vi "actuate_gapFreeExp_v0.04.vi"(0 "Phase Cluster":T3, 1 "valve Time Cluster":T2, 2 "Didn't Lift?":bool, 3 "data in":T4={"daq_ao 1"="Dev1/ao0", "daq_ai 1"="Dev1/ai0", "experiment day folder"=path "D:/DATA/8-27-15 save func testing/test.lvm", "Multiclamp init error"=0, "Multiclamp Handle Out"=0, "sampling rate (Hz)"=10000, "trial name"=""}, 5 "PhaseLetter":string, 7 "controls array in":refnum<vi>[](array[refnum]), 9 "time to wait for solution change (min)":dbl=2.5 min=0.0 step=0.01, 11 "error in":errorcluster, 12 "common cluster":T6, 13 "individual controls in":T5) -> (4 "output cluster":T1, 8 "jumptestMonitor":waveform(dbl)[](graph) caption="protocol response", 10 "control array out":refnum<vi>[](array[refnum]), 14 "experiment VI ref":refnum<vi>, 15 "error out":errorcluster)   [LabVIEW 2019]
uses:
  pipette cleaning/pressure box/cleaning_soft/controls/actuator_type.ctl
  pipette cleaning/pressure box/cleaning_soft/controls/actuator_cluster.ctl
  machine_vision/coordinate model vis/transform_properties_actuators.ctl
  machine_vision/controls/transform_cluster_actuator.ctl
  controls/NH_method.ctl
  pipette cleaning/pressure box/cleaning_soft/controls/pressure_box_type.ctl
  pipette cleaning/pressure box/cleaning_soft/controls/pressure_box_control.ctl
  multipatch/controls/multipatch_common_controls_v4.ctl
  controls/memtest_def.ctl
  multipatch/controls/multipatch_individual_controls_v5.ctl
  Controls/Data.ctl
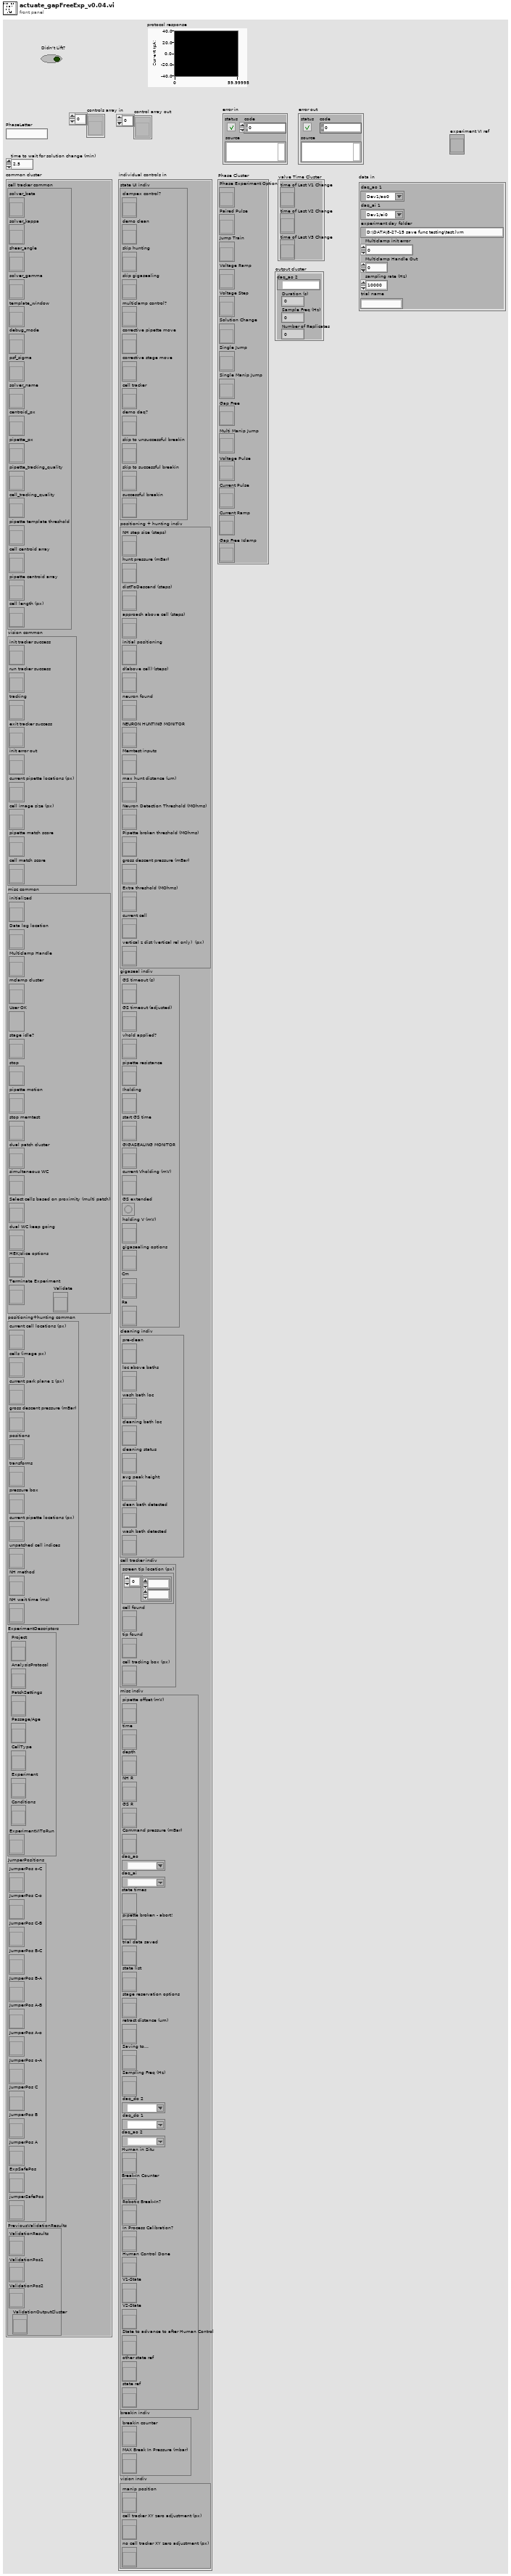
[diagram p1: front panel]
types:
  T1 = cluster{"daq_ao 2":tag, "Duration (s)":dbl, "Sample Freq (Hz)":dbl, "Number of Replicates":i16}
  T2 = cluster{"time of Last V1 Change":refnum<vi>, "time of Last V2 Change":refnum<vi>, "time of Last V3 Change":refnum<vi>}
  T3 = cluster{"Phase Experiment Option":refnum<vi>, "Paired Pulse":refnum<vi>, "Jump Train":refnum<vi>, "Voltage Ramp":refnum<vi>, "Voltage Step":refnum<vi>, "Solution Change":refnum<vi>, "Single Jump":refnum<vi>, "Single Manip Jump":refnum<vi>, "Gap Free":refnum<vi>, "Multi Manip Jump":refnum<vi>, "Voltage Pulse":refnum<vi>, "Current Pulse":refnum<vi>, "Current Ramp":refnum<vi>, "Gap Free Iclamp":refnum<vi>}
  T4 = typedef "Data.ctl" = cluster{"daq_ao 1":tag, "daq_ai 1":tag, "experiment day folder":path, "Multiclamp init error":i32, "Multiclamp Handle Out":u32, "sampling rate (Hz)":i32, "trial name":string}
  T5 = typedef "multipatch_individual_controls_v5.ctl" = cluster{"state UI indiv":cluster{"clampex control?":refnum<vi>, "demo clean":refnum<vi>, "skip hunting":refnum<vi>, "skip gigasealing":refnum<vi>, "multiclamp control?":refnum<vi>, "corrective pipette move":refnum<vi>, "corrective stage move":refnum<vi>, "cell tracker":refnum<vi>, "demo daq?":refnum<vi>, "skip to unsuccessful breakin":refnum<vi>, "skip to successful breakin":refnum<vi>, "successful breakin":refnum<vi>}, "positioning + hunting indiv":cluster{"NH step size (steps)":refnum<vi>, "hunt pressure (mBar)":refnum<vi>, "distToDescend (steps)":refnum<vi>, "approach above cell (steps)":refnum<vi>, "initial positioning":refnum<vi>, "d(above cell) (steps)":refnum<vi>, "neuron found":refnum<vi>, "NEURON HUNTING MONITOR":refnum<vi>, "Memtest inputs":refnum<vi>, "max hunt distance (um)":refnum<vi>, "Neuron Detection Threshold (MOhms)":refnum<vi>, "Pipette broken threshold (MOhms)":refnum<vi>, "gross descent pressure (mBar)":refnum<vi>, "Extra threshold (MOhms)":refnum<vi>, "current cell":refnum<vi>, "vertical z dist (vertical rel only)  (px)":refnum<vi>}, "gigaseal indiv":cluster{"GS timeout (s)":refnum<vi>, "GS timeout (adjusted)":refnum<vi>, "vhold applied?":refnum<vi>, "pipette resistance":refnum<vi>, "Iholding":refnum<vi>, "start GS time":refnum<vi>, "GIGASEALING MONITOR":refnum<vi>, "current Vholding (mV)":refnum<vi>, "GS extended":refnum<vi>, "holding V (mV)":refnum<vi>, "gigasealing options":refnum<vi>, "Cm":refnum<vi>, "Ra ":refnum<vi>}, "cleaning indiv":cluster{"pre-clean":refnum<vi>, "loc above baths":refnum<vi>, "wash bath loc":refnum<vi>, "cleaning bath loc":refnum<vi>, "cleaning status":refnum<vi>, "avg peak height":refnum<vi>, "clean bath detected":refnum<vi>, "wash bath detected":refnum<vi>}, "cell tracker indiv":cluster{"screen tip location (px)":refnum<vi>, "cell found":refnum<vi>, "tip found":refnum<vi>, "cell tracking box (px)":refnum<vi>}, "misc indiv":cluster{"pipette offset (mV)":refnum<vi>, "time":refnum<vi>, "depth":refnum<vi>, "NH R":refnum<vi>, "GS R":refnum<vi>, "Command pressure (mBar)":refnum<vi>, "daq_ao":tag, "daq_ai":tag, "state times":refnum<vi>, "pipette broken - abort!":refnum<vi>, "trial data saved":refnum<vi>, "state list":refnum<vi>, "stage reservation options":refnum<vi>, "retract distance (um)":refnum<vi>, "Saving to...":refnum<vi>, "Sampling Freq (Hz)":refnum<vi>, "daq_do 2":tag, "daq_do 1":tag, "daq_ao 2":tag, "Human in Situ":refnum<vi>, "Break-In Counter":refnum<vi>, "Robotic Break-In?":refnum<vi>, "In Process Calibration?":refnum<vi>, "Human Control Done":refnum<vi>, "V1-State":refnum<vi>, "V2-State":refnum<vi>, "State to advance to after Human Control":refnum<vi>, "other state ref":refnum<vi>, "state ref":refnum<vi>}, "breakin indiv":cluster{"breakin counter":refnum<vi>, "MAX Break In Pressure (mbar)":refnum<vi>}, "vision indiv":cluster{"manip position":refnum<vi>, "cell tracker XY zero adjustment (px)":refnum<vi>, "no cell tracker XY zero adjustment (px)":refnum<vi>}}
  T6 = typedef "multipatch_common_controls_v4.ctl" = cluster{"cell tracker common":cluster{"solver_beta":refnum<vi>, "solver_kappa":refnum<vi>, "shear_angle":refnum<vi>, "solver_gamma":refnum<vi>, "template_window":refnum<vi>, "debug_mode":refnum<vi>, "psf_sigma":refnum<vi>, "solver_name":refnum<vi>, "centroid_px":refnum<vi>, "pipette_px":refnum<vi>, "pipette_tracking_quality":refnum<vi>, "cell_tracking_quality":refnum<vi>, "pipette template threshold":refnum<vi>, "cell centroid array":refnum<vi>, "pipette centroid array":refnum<vi>, "cell length (px)":refnum<vi>}, "vision common":cluster{"init tracker success":refnum<vi>, "run tracker success":refnum<vi>, "tracking":refnum<vi>, "exit tracker success":refnum<vi>, "init error out":refnum<vi>, "current pipette locations (px)":refnum<vi>, "cell image size (px)":refnum<vi>, "pipette match score":refnum<vi>, "cell match score":refnum<vi>}, "misc common":cluster{"initialized":refnum<vi>, "Data log location":refnum<vi>, "Multiclamp Handle":refnum<vi>, "mclamp cluster":refnum<vi>, "User OK":refnum<vi>, "stage idle?":refnum<vi>, "stop":refnum<vi>, "pipette motion":refnum<vi>, "stop memtest":refnum<vi>, "dual patch cluster":refnum<vi>, "simultaneous WC":refnum<vi>, "Select cells based on proximity (multi patch)":refnum<vi>, "dual WC keep going":refnum<vi>, "HEK/slice options":refnum<vi>, "Terminate Experiment":refnum<vi>, "Validate":refnum<vi>}, "positioning+hunting common":cluster{"current cell locations (px)":refnum<vi>, "cells (image px)":refnum<vi>, "current park plane z (px)":refnum<vi>, "gross descent pressure (mBar)":refnum<vi>, "positions":refnum<vi>, "transforms":refnum<vi>, "pressure box":refnum<vi>, "current pipette locations (px)":refnum<vi>, "unpatched cell indices":refnum<vi>, "NH method":refnum<vi>, "NH wait time (ms)":refnum<vi>}, "ExperimentDescriptors":cluster{"Project":refnum<vi>, "AnalysisProtocol":refnum<vi>, "PatchSettings":refnum<vi>, "Passage/Age":refnum<vi>, "CellType":refnum<vi>, "Experiment":refnum<vi>, "Conditions":refnum<vi>, "ExperimentVIToRun":refnum<vi>}, "JumperPositions":cluster{"JumperPos o-C":refnum<vi>, "JumperPos C-o":refnum<vi>, "JumperPos C-B":refnum<vi>, "JumperPos B-C":refnum<vi>, "JumperPos B-A":refnum<vi>, "JumperPos A-B":refnum<vi>, "JumperPos A-o":refnum<vi>, "JumperPos o-A":refnum<vi>, "JumperPos C":refnum<vi>, "JumperPos B":refnum<vi>, "JumperPos A":refnum<vi>, "ExpSafePos":refnum<vi>, "jumperSafePos":refnum<vi>}, "PreviousValidationResults":cluster{"ValidationResults":refnum<vi>, "ValidationPos1":refnum<vi>, "ValidationPos2":refnum<vi>, "ValidationOutputCluster":refnum<vi>}}
  T7 = cluster{"Which Position to use for Experiment":enum16{"Jumper Safe Position", "Experiment Safe Position", "Jumper Position A", "Jumper Position B", "Jumper Position C", "Jumper Position o-A", "Jumper Position A-o", "Jumper Position A-B", "Jumper Position B-A", "Jumper Position B-C", "Jumper Position C-B", "Jumper Position C-o", "Jumper Position o-C", "Don't Move"}, "Duration (s)":dbl, "Valve 1 Position":i16, "Valve 2 Position":i16, "Replicates":dbl, "Vholding (mV)":dbl, "Valve 3 Position":i16, "valve 1 used now?":bool, "valve 2 used now?":bool, "valve 3 used now? ":bool, "Record During Solution Change?":bool}
  T8 = enum16{"Jumper Safe Position", "Experiment Safe Position", "Jumper Position A", "Jumper Position B", "Jumper Position C", "Jumper Position o-A", "Jumper Position A-o", "Jumper Position A-B", "Jumper Position B-A", "Jumper Position B-C", "Jumper Position C-B", "Jumper Position C-o", "Jumper Position o-C", "Don't Move"}
  T9 = enum16{"manipulator 1", "manipulator 2", "manipulator 3", "manipulator 4"}
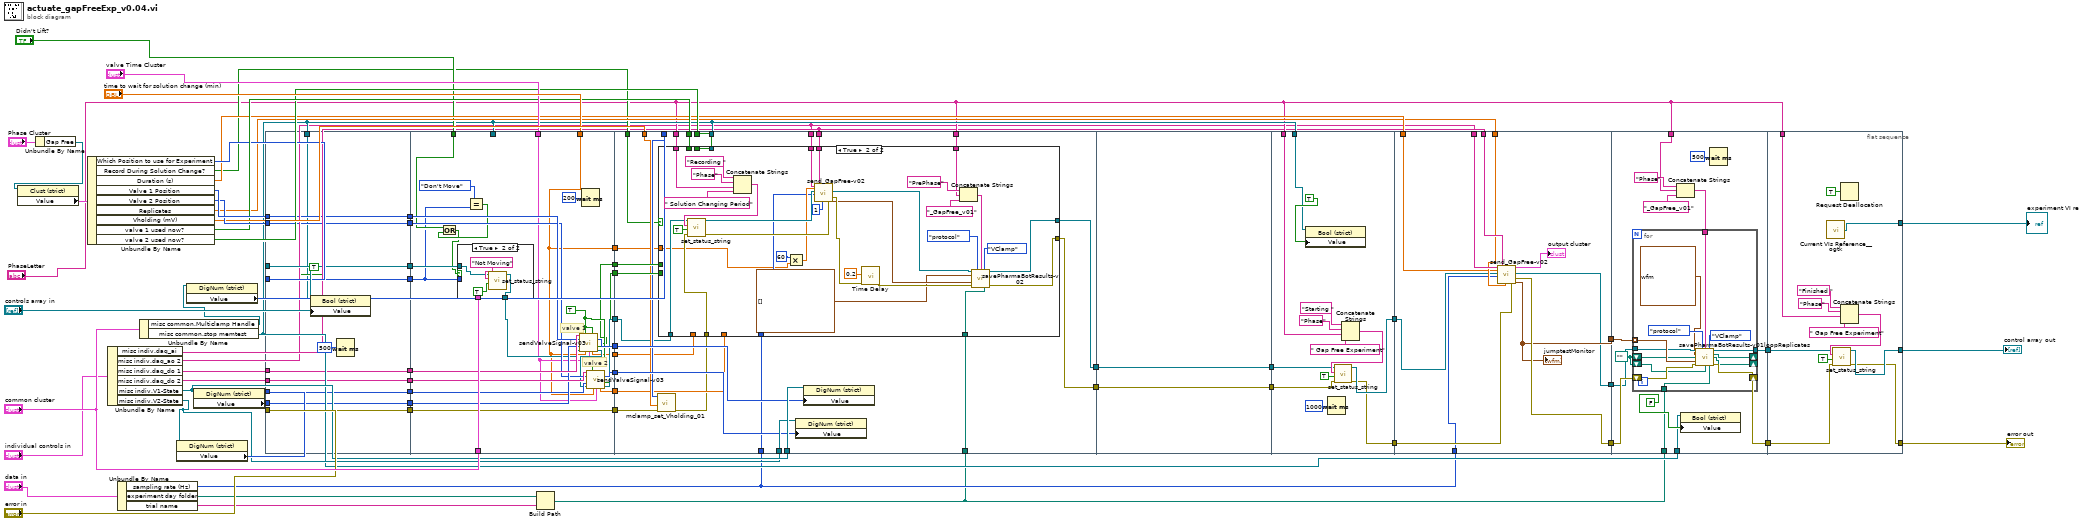
[diagram p0: block diagram]
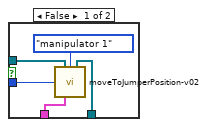
[diagram p2: hidden frame]
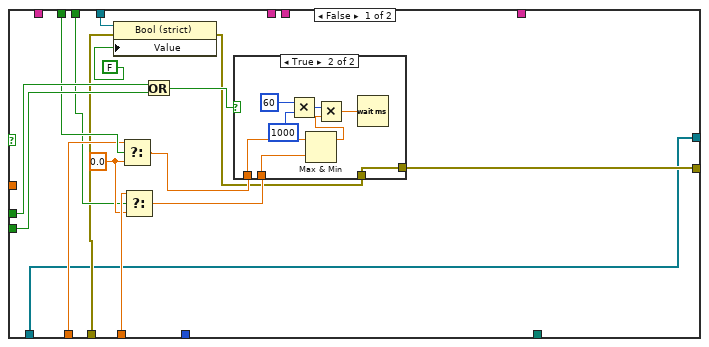
[diagram p3: hidden frame]
diagram:
  n1 = Unbundle By Name("Phase Cluster") -> ("Gap Free"=w50:refnum<vi>)
  n2 = property class="Clust (strict)"(reference=w50) -> ("Value"=w49:T7)  [unwired: 1 in, 2 out]
  n3 = Unbundle By Name(w49) -> ("Which Position to use for Experiment"=w30:T8, "Record During Solution Change?"=w17:bool, "Duration (s)"=w29:dbl, "Valve 1 Position"=w48:i16, "Valve 2 Position"=w47:i16, "Replicates"=w28:dbl, "Vholding (mV)"=w38:dbl, "valve 1 used now?"=w32:bool, "valve 2 used now?"=w31:bool)
  n4 = Unbundle By Name("individual controls in") -> ("misc indiv.daq_ai"=w14:tag, "misc indiv.daq_ao 2"=w13:tag, "misc indiv.daq_do 1"=w66:tag, "misc indiv.daq_do 2"=w65:tag, "misc indiv.V1-State"=w58:refnum<vi>, "misc indiv.V2-State"=w57:refnum<vi>)
  n5 = Unbundle By Name("data in") -> ("sampling rate (Hz)"=w12:i32, "experiment day folder"=w53:path, "trial name"=w52:string)
  n6 = Unbundle By Name("common cluster") -> ("misc common.Multiclamp Handle"=w11:refnum<vi>, "misc common.stop memtest"=w16:refnum<vi>)
  n7 = property class="DigNum (strict)"(reference=w57) -> ("Value"=w59:u16)  [unwired: 1 in, 2 out]
  n8 = property class="DigNum (strict)"(reference=w11) -> ("Value"=w37:u32)  [unwired: 1 in, 2 out]
  n9 = property class="DigNum (strict)"(reference=w58) -> ("Value"=w60:u16)  [unwired: 1 in, 2 out]
  n10 = flat-sequence {
    tunnel: "controls array in" -> [w72]
    tunnel: w47 -> [w73]
    tunnel: w48 -> [w74]
    tunnel: w59 -> [w75]
    tunnel: w60 -> [w76]
    tunnel: "error in" -> [w77]
    tunnel: w65 -> [w78]
    tunnel: w66 -> [w79]
    tunnel: w30 -> [w80]
    tunnel: [w80] -> w26
    tunnel: [w79] -> w25
    tunnel: [w78] -> w24
    tunnel: [w77] -> w23
    tunnel: [w76] -> w22
    tunnel: [w75] -> w21
    tunnel: [w74] -> w20
    tunnel: [w73] -> w19
    tunnel: [w72] -> w18
    tunnel: w16 -> [w70]
    tunnel: "common cluster" -> [w107]
    tunnel: [w104] -> w62
    tunnel: [w101] -> w56
    tunnel: [w100] -> w55
    tunnel: [w94] -> w44
    tunnel: [w92] -> w40
    tunnel: [w91] -> w39
    tunnel: "time to wait for solution change (min)" -> [w81]
    tunnel: "valve Time Cluster" -> [w90]
    tunnel: [w89] -> w34
    tunnel: [w88] -> w33
    tunnel: w26 -> [w84]
    tunnel: w25 -> [w106]
    tunnel: w24 -> [w105]
    tunnel: w23 -> [w104]
    tunnel: w22 -> [w103]
    tunnel: w21 -> [w102]
    tunnel: w20 -> [w99]
    tunnel: w19 -> [w98]
    tunnel: w18 -> [w97]
    tunnel: w16 -> [_]
    tunnel: "Didn't Lift?" -> [w86]
    tunnel: [w81] -> w9
    tunnel: w62 -> [w135]
    tunnel: w58 -> [w142]
    tunnel: w57 -> [w141]
    tunnel: w56 -> [w140]
    tunnel: w55 -> [w139]
    tunnel: w44 -> [w125]
    tunnel: w40 -> [w138]
    tunnel: w39 -> [w137]
    tunnel: w38 -> [w136]
    tunnel: w37 -> [w134]
    tunnel: w34 -> [w132]
    tunnel: w33 -> [w131]
    tunnel: w32 -> [w133]
    tunnel: [w130] -> _
    tunnel: w31 -> [w130]
    tunnel: w17 -> [w129]
    tunnel: w16 -> [w127]
    tunnel: "PhaseLetter" -> [w126]
    tunnel: "PhaseLetter" -> [w124]
    tunnel: [w123] -> w8
    tunnel: [w122] -> w6
    tunnel: w14 -> [w121]
    tunnel: w13 -> [w120]
    tunnel: w12 -> [w119]
    tunnel: w10 -> [w118]
    tunnel: w9 -> [w117]
    tunnel: w8 -> [w201]
    tunnel: [w201] -> w7
    tunnel: w6 -> [w200]
    tunnel: [w200] -> w5
    tunnel: w16 -> [w204]
    tunnel: [w206] -> w63
    tunnel: [w207] -> w45
    tunnel: "PhaseLetter" -> [w208]
    tunnel: w7 -> [w203]
    tunnel: w5 -> [w202]
    tunnel: w14 -> [w225]
    tunnel: w13 -> [w224]
    tunnel: w63 -> [w220]
    tunnel: [w218] -> w3
    tunnel: w28 -> [w222]
    tunnel: w29 -> [w221]
    tunnel: w12 -> [w215]
    tunnel: [w219] -> w2
    tunnel: [w216] -> w1
    tunnel: w45 -> [w217]
    tunnel: w16 -> [w238]
    tunnel: w3 -> [w237]
    tunnel: w10 -> [w236]
    tunnel: "PhaseLetter" -> [w227]
    tunnel: w2 -> [w232]
    tunnel: w1 -> [w231]
    tunnel: [w229] -> w42
    tunnel: [w230] -> w41
    tunnel: [w259] -> w43
    tunnel: [w258] -> w61
    tunnel: w42 -> [w257]
    tunnel: w41 -> [w260]
    tunnel: "PhaseLetter" -> [w256]
    tunnel: [w255] -> w4
    frame #0 {
      n11 = property class="Bool (strict)"(reference=w70, "Value"=TRUE ("stop memtest")) -> ()  [unwired: 1 in, 2 out]
      n12 = Wait (ms)(milliseconds to wait=u32 500) -> ()  [unwired: 1 out]
    }
    frame #1 {
      w93 = TRUE ("Set Status")
      # "valve 2"
      # "valve 1"
      n13 = Equal?(x=T8."Don't Move" ("Which Position to use for Experiment"), y=w84) -> (x = y?=w83:bool)
      n14 = Or(x=w86, y=w83) -> (x .or. y?=w82:bool)
      n15 = case shown="True" w82 {
        tunnel: w84 -> [w112 _]
        tunnel: w107 -> [w111 _]
        tunnel: w97 -> [w109 w113]
        tunnel: [w108 w114] -> w96
        frame False {
          n16 = call "moveToJumperPosition-v02.vi"("which manipulator"=T9."manipulator 1", "controls array in"=w109, "Which Jumper Position to move to?"=w112, "common cluster"=w111) -> ("control array out"=w108:refnum<vi>[])  [unwired: 10 in, 1 out]
        }
        frame True {
          n17 = call "set_status_string.vi"("new line?"=TRUE, "status string in"="Not Moving", "controls array"=w113) -> ("controls array out"=w114:refnum<vi>[])  [unwired: 7 in, 1 out]
        }
      }
      n18 = call "sendValveSignal-v03.vi"("daq_do"=w106, "Set Status"=w93, "Valve1?"=w93, "ChangeToValve"=w99, "CurrentValve"=w103, "controls array in"=w96, "time to wait for solution change (min)"=w81, "valve Time Cluster"=w90) -> ("ValveSetTo"=w100:u16, "valve changed?"=w92:bool, "additional time to wait (min)"=w89:dbl, "control array out"=w95:refnum<vi>[])  [unwired: 4 in]
      n19 = Wait (ms)(milliseconds to wait=u32 200) -> ()  [unwired: 1 out]
      n20 = call "sendValveSignal-v03.vi"("daq_do"=w105, "Set Status"=w93, "ChangeToValve"=w98, "CurrentValve"=w102, "controls array in"=w95, "time to wait for solution change (min)"=w81, "valve Time Cluster"=w90) -> ("ValveSetTo"=w101:u16, "valve changed?"=w91:bool, "additional time to wait (min)"=w88:dbl, "control array out"=w94:refnum<vi>[])  [unwired: 5 in]
    }
    frame #2 {
      n21 = call "mclamp_set_Vholding_01.vi"("error in (no error)"=w135, "set holding (mV)"=w136, "Multiclamp Handle Out"=w134) -> ("error out"=w128:errorcluster)  [unwired: 7 in, 1 out]
      n22 = case shown="True" w129 {
        tunnel: w138 -> [w157 _]
        tunnel: w137 -> [w156 _]
        tunnel: w133 -> [w154 _]
        tunnel: w132 -> [w153 _]
        tunnel: w131 -> [w152 _]
        tunnel: w130 -> [w149 _]
        tunnel: w128 -> [w145 w193]
        tunnel: [w148 w184] -> w122
        tunnel: w127 -> [w146 _]
        tunnel: w126 -> [_ w195]
        tunnel: w125 -> [w143 w194]
        tunnel: [w143 w182] -> w123
        tunnel: w124 -> [_ w183]
        tunnel: w121 -> [_ w181]
        tunnel: w120 -> [_ w180]
        tunnel: w119 -> [_ w174]
        tunnel: w118 -> [_ w173]
        tunnel: w117 -> [_ w169]
        frame False {
          w150 = 0.0 ("f")
          n23 = property class="Bool (strict)"(reference=w146, error in=w145, "Value"=FALSE ("stop memtest")) -> (error out=w144:errorcluster)  [unwired: 1 out]
          n24 = Select(t=w153, s=w154, f=w150) -> (s? t:f=w155:dbl)
          n25 = Select(t=w152, s=w149, f=w150) -> (s? t:f=w151:dbl)
          n26 = Or(x=w157, y=w156) -> (x .or. y?=w158:bool)
          n27 = case shown="True" w158 {
            tunnel: w155 -> [_ w163]
            tunnel: w151 -> [_ w162]
            tunnel: [w159 w160] -> w148
            tunnel: w144 -> [w159 w160]
            frame False {
            }
            frame True {
              n28 = Multiply(x=u32 60 ("milliseconds to wait"), y=u32 1000) -> (x*y=w165:u32)
              n29 = Max & Min(x=w163, y=w162) -> (max(x,y)=w161:dbl)  [unwired: 1 out]
              n30 = Multiply(x=w165, y=w161) -> (x*y=w164:dbl)
              n31 = Wait (ms)(milliseconds to wait=w164) -> ()  [unwired: 1 out]
            }
          }
        }
        frame True {
          n32 = Concatenate Strings("Recording " ("string"), "Phase" ("string"), w195, " Solution Changing Period" ("string")) -> (w198:string)
          n33 = call "set_status_string.vi"("error in"=w193, "new line?"=TRUE, "status string in"=w198, "controls array"=w194) -> ("error out"=w191:errorcluster, "controls array out"=w179:refnum<vi>[])  [unwired: 6 in]
          n34 = Multiply(x=u32 60 ("milliseconds to wait"), y=w169) -> (x*y=w175:dbl)
          n35 = call "send_GapFree-v02.vi"("daq_ao 2"=w180, "Duration (s)"=w175, "controls array in"=w179, "Sample Freq (Hz)"=w174, "daq_ai"=w181, "Number of Replicates"=i16 1, "error in"=w191) -> ("control array out"=w178:refnum<vi>[], "error out"=w185:errorcluster, "jumptestMonitor"=w170:waveform(dbl)[])  [unwired: 8 in, 2 out]
          n36 = call "Time Delay"("error in (no error)"=w185, "Delay Time (s)"=0.2) -> ("error out"=w172:errorcluster)  [unwired: 9 in]
          n37 = Concatenate Strings("PrePhase" ("string"), w183, "_GapFree_v01" ("string")) -> (w188:string)
          n38 = call "savePharmaBotResults-v02.vi"("controls array"=w178, "protocol or memtest"=enum16{"protocol", "memtest", "validation"}."protocol", "ExpPhase"=w188, "which clamp"=enum16{"VClamp", "IClamp"}."VClamp", "protocol waveform"=waveform(dbl)[] [] ("appended array"), "protocol response"=w170, "error in"=w172, "Save to (folder dir)"=w173) -> ("controls array out"=w182:refnum<vi>[], "error out"=w184:errorcluster)  [unwired: 6 in]
        }
      }
      n39 = property class="DigNum (strict)"(reference=w141, "Value"=w140) -> ()  [unwired: 1 in, 2 out]
      n40 = property class="DigNum (strict)"(reference=w142, "Value"=w139) -> ()  [unwired: 1 in, 2 out]
    }
    frame #3 {
    }
    frame #4 {
      n41 = property class="Bool (strict)"(reference=w204, "Value"=TRUE ("stop memtest")) -> ()  [unwired: 1 in, 2 out]
      n42 = Wait (ms)(milliseconds to wait=u32 1000) -> ()  [unwired: 1 out]
      n43 = Concatenate Strings("Starting " ("string"), "Phase" ("string"), w208, " Gap Free Experiment" ("string")) -> (w210:string)
      n44 = call "set_status_string.vi"("error in"=w202, "new line?"=TRUE, "status string in"=w210, "controls array"=w203) -> ("error out"=w206:errorcluster, "controls array out"=w207:refnum<vi>[])  [unwired: 6 in]
    }
    frame #5 {
      n45 = call "send_GapFree-v02.vi"("daq_ao 2"=w224, "Duration (s)"=w221, "controls array in"=w217, "Sample Freq (Hz)"=w215, "daq_ai"=w225, "Number of Replicates"=w222, "error in"=w220) -> ("output cluster"=→"output cluster":T1, "control array out"=w216:refnum<vi>[], "error out"=w219:errorcluster, "jumptestMonitor"=w218:waveform(dbl)[])  [unwired: 8 in, 1 out]
      "jumptestMonitor" <- w218
    }
    frame #6 {
      w226 = path "" ("rec path out")
      n46 = Concatenate Strings("Phase" ("string"), w227, "_GapFree_v01" ("string")) -> (w235:string)
      n47 = for {
        tunnel: w237 -> [w253] mode=indexing
        tunnel: w236 -> [w250]
        tunnel: w235 -> [w249]
        tunnel: w231 -> [w247]
        tunnel: [w246] -> w230
        shift-right: [w245] -> w229
        shift-left: w232 -> [w248]
        shift-right: [w243] -> _
        shift-left: w226 -> [w240]
        shift-right: [w242] -> _
        shift-left: w226 -> [w241]
        n48 = call "savePharmaBotResults-v01loopReplicates.vi"("controls array"=w247, "protocol or memtest"=enum16{"protocol", "memtest", "validation"}."protocol", "ExpPhase"=w249, "which clamp"=enum16{"VClamp", "IClamp"}."VClamp", "protocol waveform"=waveform(dbl) {"t0"=timestamp(0 s since 1904-01-01), "dt"=1.0, "Y"=[]}, "loop rec path in"=w240, "protocol response"=w253, "error in"=w248, "loop wave path in 2"=w241, "Save to (folder dir)"=w250) -> ("controls array out"=w246:refnum<vi>[], "rec path out"=w243:path, "wave path out 2"=w242:path, "error out"=w245:errorcluster)  [unwired: 2 in]
      }
      n49 = property class="Bool (strict)"(reference=w238, "Value"=FALSE ("stop memtest")) -> ()  [unwired: 1 in, 2 out]
      n50 = Wait (ms)(milliseconds to wait=u32 500) -> ()  [unwired: 1 out]
    }
    frame #7 {
      n51 = call "Current VIs Reference__ogtk.vi"() -> ("Current VI's reference"=w255:refnum<vi>)  [unwired: 5 in]
      n52 = Concatenate Strings("Finished " ("string"), "Phase" ("string"), w256, " Gap Free Experiment" ("string")) -> (w262:string)
      n53 = call "set_status_string.vi"("error in"=w257, "new line?"=TRUE, "status string in"=w262, "controls array"=w260) -> ("error out"=w258:errorcluster, "controls array out"=w259:refnum<vi>[])  [unwired: 6 in]
      n54 = Request Deallocation(TRUE ("flag")) -> ()
    }
  }
  n55 = Build Path(base path=w53, name or relative path=w52) -> (appended path=w10:path)
  "error out" <- w61
  "control array out" <- w43
  "experiment VI ref" <- w4
